vi "保存数据.vi"(0 "数据":sgl[][](array[numeric]), 3 "引用句柄输出":refnum<file>) -> ()   [LabVIEW 2016]
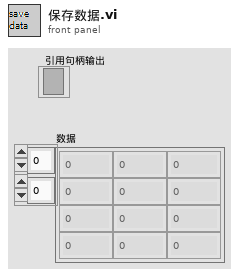
[diagram p1: front panel]
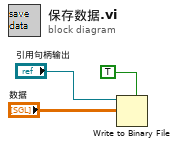
[diagram p0: block diagram]
diagram:
  n1 = Write to Binary File(file (use dialog)="引用句柄输出", data="数据", 5:TRUE ("预置数组或字符串大小？(T)")) -> ()  [unwired: 3 in, 3 out]
